vi "Generate SN.vi"(8 "error in (no error)":errorcluster caption="entrée d'erreur (pas d'erreur)", 11 "Firebase Recovery_SN en entrée":refnum<class "Firebase Recovery_SN.lvclass">) -> (0 "error out":errorcluster caption="sortie d'erreur", 3 "Firebase Recovery_SN en sortie":refnum<class "Firebase Recovery_SN.lvclass">)   [LabVIEW 2020, in "Library Instrument & Equipement.lvlib" / "Library FireBase.lvlib" / "Firebase Recovery_SN.lvclass"]
uses:
  Firebase Recovery_SN.lvclass
  C:/Users/ngarcin/OneDrive - Altyor/Standard TB/Class/Firebase/Source/Firebase Driver/Firebase Driver.lvclass
  Firebase Recovery_SN.lvclass/Firebase Recovery_SN.ctl
  JSON API/JSON Value/Set from JSON string.vi
  JSON API/JSON Value/JSON Value.lvclass
  Commun VI/Library Commun.lvlib
  JSON API/Variant JSON/Variant JSON.lvlib
  JSON API/Get Polymorphic/JSON GetSet.lvlib
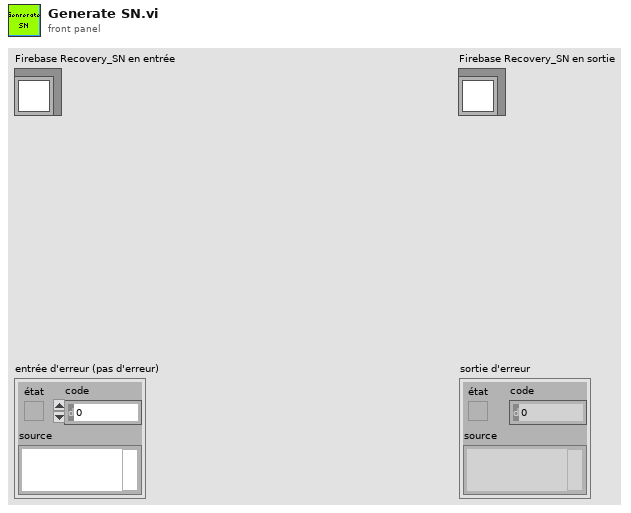
[diagram p1: front panel]
types:
  T1 = cluster{"fields":cluster{"Value":cluster{"stringValue":string}}}
  T2 = cluster{"document":cluster{"name":string, "fields":cluster{"Value":cluster{"stringValue":string}}}}[]
  T3 = cluster{"document":cluster{"name":string, "fields":cluster{"Value":cluster{"stringValue":string}}}}
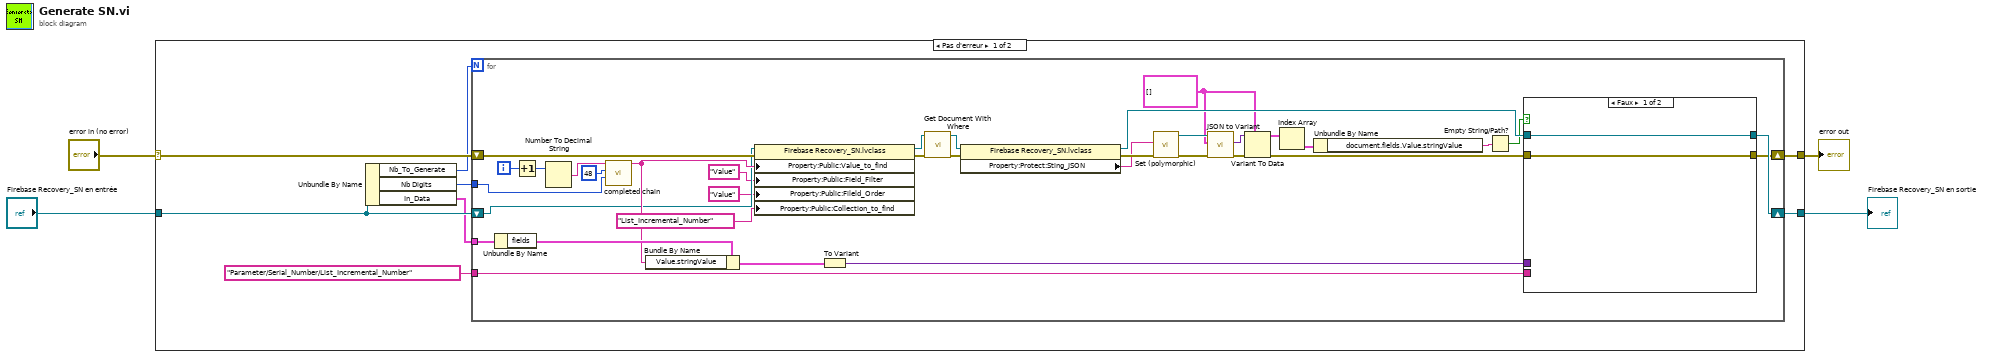
[diagram p0: block diagram]
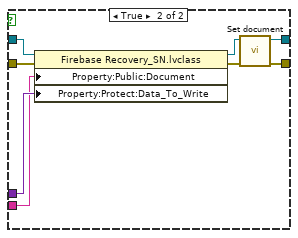
[diagram p2: hidden frame]
diagram:
  n1 = case shown="Pas d'erreur" "error in (no error)" {
    selector: "error in (no error)" -> [w10 w59]
    tunnel: [w9 w59] -> w3
    tunnel: [w11 w58] -> w1
    tunnel: "Firebase Recovery_SN en entrée" -> [w8 w58]
    frame No Error {
      n2 = Unbundle By Name(w8) -> ("Nb_To_Generate"=w6:u16, "Nb Digits"=w5:u8, "In_Data"=w7:T1)
      n3 = for {
        N: w6 -> [_]
        tunnel: "Parameter/Serial_Number/List_Incremental_Number" ("Collection_to_find") -> [w35]
        shift-right: [w46] -> w9
        shift-left: w10 -> [w37]
        shift-right: [w47] -> w11
        shift-left: w8 -> [w33]
        tunnel: w7 -> [w44]
        tunnel: w5 -> [w13]
        i -> [w42]
        w21 = T2 [] ("Data")
        n4 = Unbundle By Name(w44) -> ("fields"=w38:cluster{"Value":cluster{"stringValue":string}})
        n5 = Increment(x=w42) -> (x+1=w39:i32)
        n6 = Number To Decimal String(number=w39) -> (decimal integer string=w41:string)  [unwired: 1 in]
        n7 = call "completed chain.vi"("longueur"=w13, "Combler par"=u8 48, "Chaine"=w41) -> ("chaîne"=w34:string)  [unwired: 8 in]
        n8 = Bundle By Name(cluster=w38, "Value.stringValue"=w34) -> (w43:cluster{"Value":cluster{"stringValue":string}})
        n9 = property class="Firebase Recovery_SN.lvclass"(reference=w33, error in=w37, "Property:Public:Value_to_find"=w34, "Property:Public:Field_Filter"="Value" ("Field_Filter"), "Property:Public:Fileld_Order"="Value" ("Value_to_find"), "Property:Public:Collection_to_find"="List_Incremental_Number" ("Collection_to_find")) -> (reference out=w22:refnum<class "Firebase Recovery_SN.lvclass">, error out=w36:errorcluster)
        n10 = To Variant(anything=w43) -> (Variant=w45:variant)
        n11 = call-dynamic "Get Document With Where.vi"("error in (no error)"=w36, "Firebase (Default) en entrée"=w22) -> ("error out"=w26:errorcluster, "Firebase (Default) en sortie"=w25:refnum<class "Firebase Recovery_SN.lvclass">)  [unwired: 8 in]
        n12 = property class="Firebase Recovery_SN.lvclass"(reference=w25, error in=w26) -> (reference out=w23:refnum<class "Firebase Recovery_SN.lvclass">, error out=w28:errorcluster, "Property:Protect:Sting_JSON"=w27:string)
        n13 = call-poly "Set (polymorphic).vi"("error in (no error)"=w28, "JSON stream"=w27) -> ("error out"=w29:errorcluster, "JSON Value out"=w32:refnum<class "JSON Value.lvclass">)  [unwired: 7 in, 1 out]
        n14 = call "JSON to Variant.vi"("error in (no error)"=w29, "Variant (Data Type)"=w21, "JSON Value"=w32) -> ("error out"=w30:errorcluster, "Variant out"=w31:variant)  [unwired: 7 in]
        n15 = Variant To Data(error in=w30, type=w21, Variant=w31) -> (data=w17:T2, error out=w24:errorcluster)
        n16 = Index Array(array=w17) -> (element=w16:T3)  [unwired: 1 in]
        n17 = Unbundle By Name(w16) -> ("document.fields.Value.stringValue"=w15:string)
        n18 = Empty String/Path?(string/path=w15) -> (empty?=w14:bool)
        n19 = case shown="Faux" w14 {
          tunnel: [w48 w55] -> w47
          tunnel: [w49 w54] -> w46
          tunnel: w45 -> [_ w53]
          tunnel: w35 -> [_ w52]
          tunnel: w24 -> [w49 w51]
          tunnel: w23 -> [w48 w50]
          frame False {
          }
          frame True {
            n20 = property class="Firebase Recovery_SN.lvclass"(reference=w50, error in=w51, "Property:Public:Document"=w52, "Property:Protect:Data_To_Write"=w53) -> (reference out=w57:refnum<class "Firebase Recovery_SN.lvclass">, error out=w56:errorcluster)
            n21 = call-dynamic "Set document.vi"("error in (no error)"=w56, "Firebase (Default) en entrée"=w57) -> ("error out"=w54:errorcluster, "Firebase (Default) en sortie"=w55:refnum<class "Firebase Recovery_SN.lvclass">)  [unwired: 8 in]
          }
        }
      }
    }
    frame Error {
    }
  }
  "error out" <- w3
  "Firebase Recovery_SN en sortie" <- w1
